vi "2 polar_v_plot.vi"(1 "Wind Vector":cluster{"Wind R":dbl, "Wind Theta":dbl}, 2 "Boat Angle":dbl) -> (0 "Velocity":dbl)   [LabVIEW 2011]
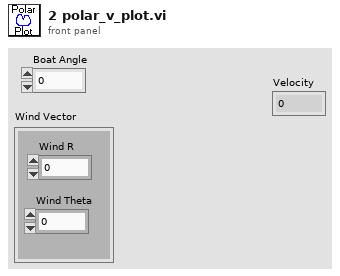
[diagram p1: front panel]
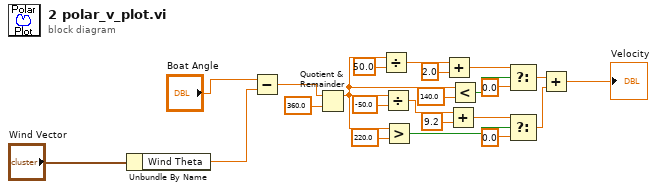
[diagram p0: block diagram]
diagram:
  n1 = Unbundle By Name("Wind Vector") -> ("Wind Theta"=w19:dbl)
  n2 = Subtract(x="Boat Angle", y=w19) -> (x-y=w22:dbl)
  n3 = Quotient & Remainder(x=w22, y=360.0) -> (x-y*floor(x/y)=w2:dbl)  [unwired: 1 out]
  n4 = Divide(x=w2, y=50.0) -> (x/y=w10:dbl)
  n5 = Divide(x=w2, y=-50.0) -> (x/y=w5:dbl)
  n6 = Greater?(x=w2, y=220.0) -> (0:w13:bool)
  n7 = Add(x=w10, y=2.0) -> (x+y=w11:dbl)
  n8 = Add(x=w5, y=9.2) -> (x+y=w3:dbl)
  n9 = Less?(x=w2, y=140.0) -> (x < y?=w17:bool)
  n10 = Select(t=w11, s=w17, f=0.0) -> (s? t:f=w8:dbl)
  n11 = Select(t=w3, s=w13, f=0.0) -> (s? t:f=w7:dbl)
  n12 = Add(x=w8, y=w7) -> (x+y=→"Velocity":dbl)
